vi "Problem 26.vi"() -> ()   [LabVIEW 2013, in "Problem 26.lvlib"]
uses:
  Problem 26.lvlib
panel:
  in  "d":i32=7
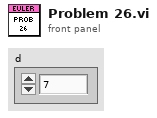
[diagram p1: front panel]
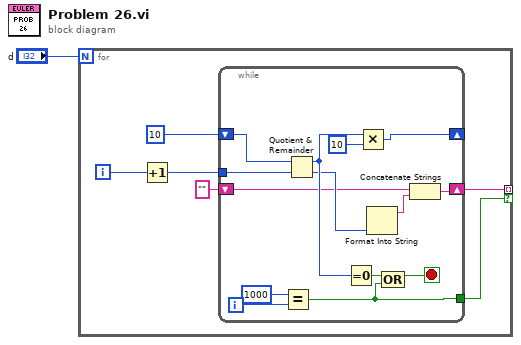
[diagram p0: block diagram]
diagram:
  n1 = for {
    N: "d" -> [_]
    tunnel: [w4] -> _ mode=indexing if=w3
    i -> [w7]
    n2 = Increment(x=w7) -> (x+1=w5:i32)
    n3 = while {
      shift-right: [w19] -> _
      shift-left: 10 ("x") -> [w20]
      tunnel: w5 -> [w21]
      tunnel: [w12] -> w3
      shift-right: [w9] -> w4
      shift-left: "" -> [w8]
      i -> [w14]
      stop <- w15 stop-if-true
      n4 = Equal?(x=1000, y=w14) -> (x = y?=w12:bool)
      n5 = Quotient & Remainder(x=w20, y=w21) -> (x-y*floor(x/y)=w17:i32, floor(x/y)=w11:i32)
      n6 = Equal To 0?(x=w17) -> (x = 0?=w16:bool)
      n7 = Multiply(x=w17, y=10) -> (x*y=w19:i32)
      n8 = Format Into String(w11) -> (resulting string=w10:string)  [unwired: 3 in, 1 out]
      n9 = Compound Arithmetic op=OR(w16, w12) -> (w15:bool)
      n10 = Concatenate Strings(w8, w10) -> (w9:string)
    }
  }
